vi "WT210 IEC 2015 Setup.vi"(0 "VISA Input":refnum<visa-resource-name>, 5 "V Range (6: 600V)":u16(ring)=4 items=["Auto", "15V", "30V", "60V", "150V", "300V", "600V"], 7 "A Range (12: 20A)":u16(ring)=10 items=["Auto", "5mA", "10mA", "20mA", "50mA", "100mA", "200mA", "0.5A", "1A", "2A", "5A", "10A", "20A", "50mV", "100mV", "200mV", "2.5V", "5V", "10V"], 11 "error in (no error)":errorcluster) -> (2 "VTHD":sgl format="%.3g", 4 "VISA Output":refnum<visa-resource-name>, 6 "Header File":string[][](array[string]), 15 "error out":errorcluster)   [LabVIEW 2016]
uses:
  <vilib>/Utility/error.llb/whitespace.ctl
  Yokogawa WT200 Series.lvlib
panel:
  in  "Tab Control":enum32{"Main", "Debug"}(tab)
  out "Sample Rate (1: 0.25s)":u16(ring)=1 items=["0.1s", "0.25s", "0.5s", "1s", "2s", "5s"]
  out "Sample Rate":string
  out "V Range":string
  out "A Range":string
  out "Instrument ID":string
  out "Date & Time":string
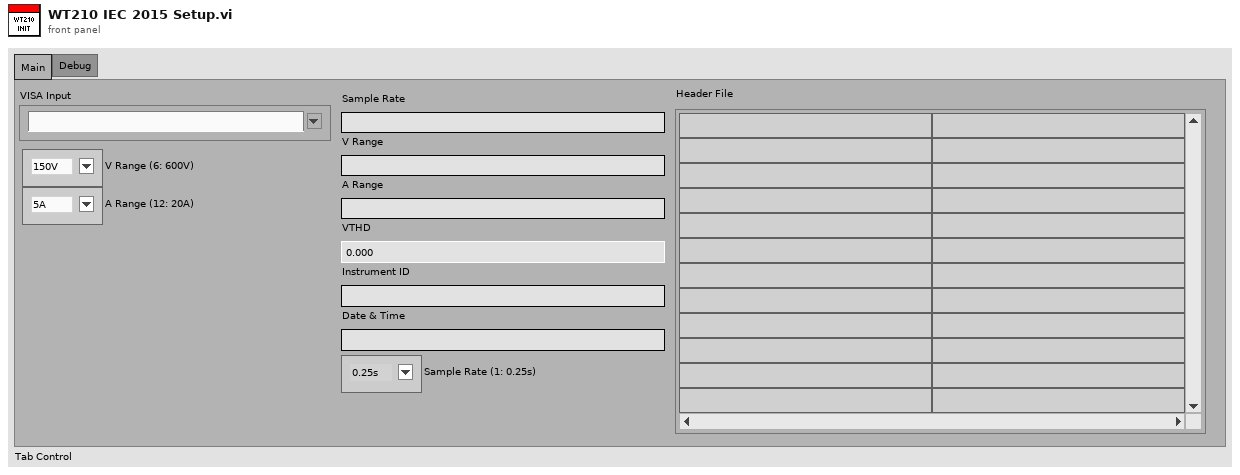
[diagram p1: front panel]
types:
  T1 = typedef "whitespace.ctl" = u16
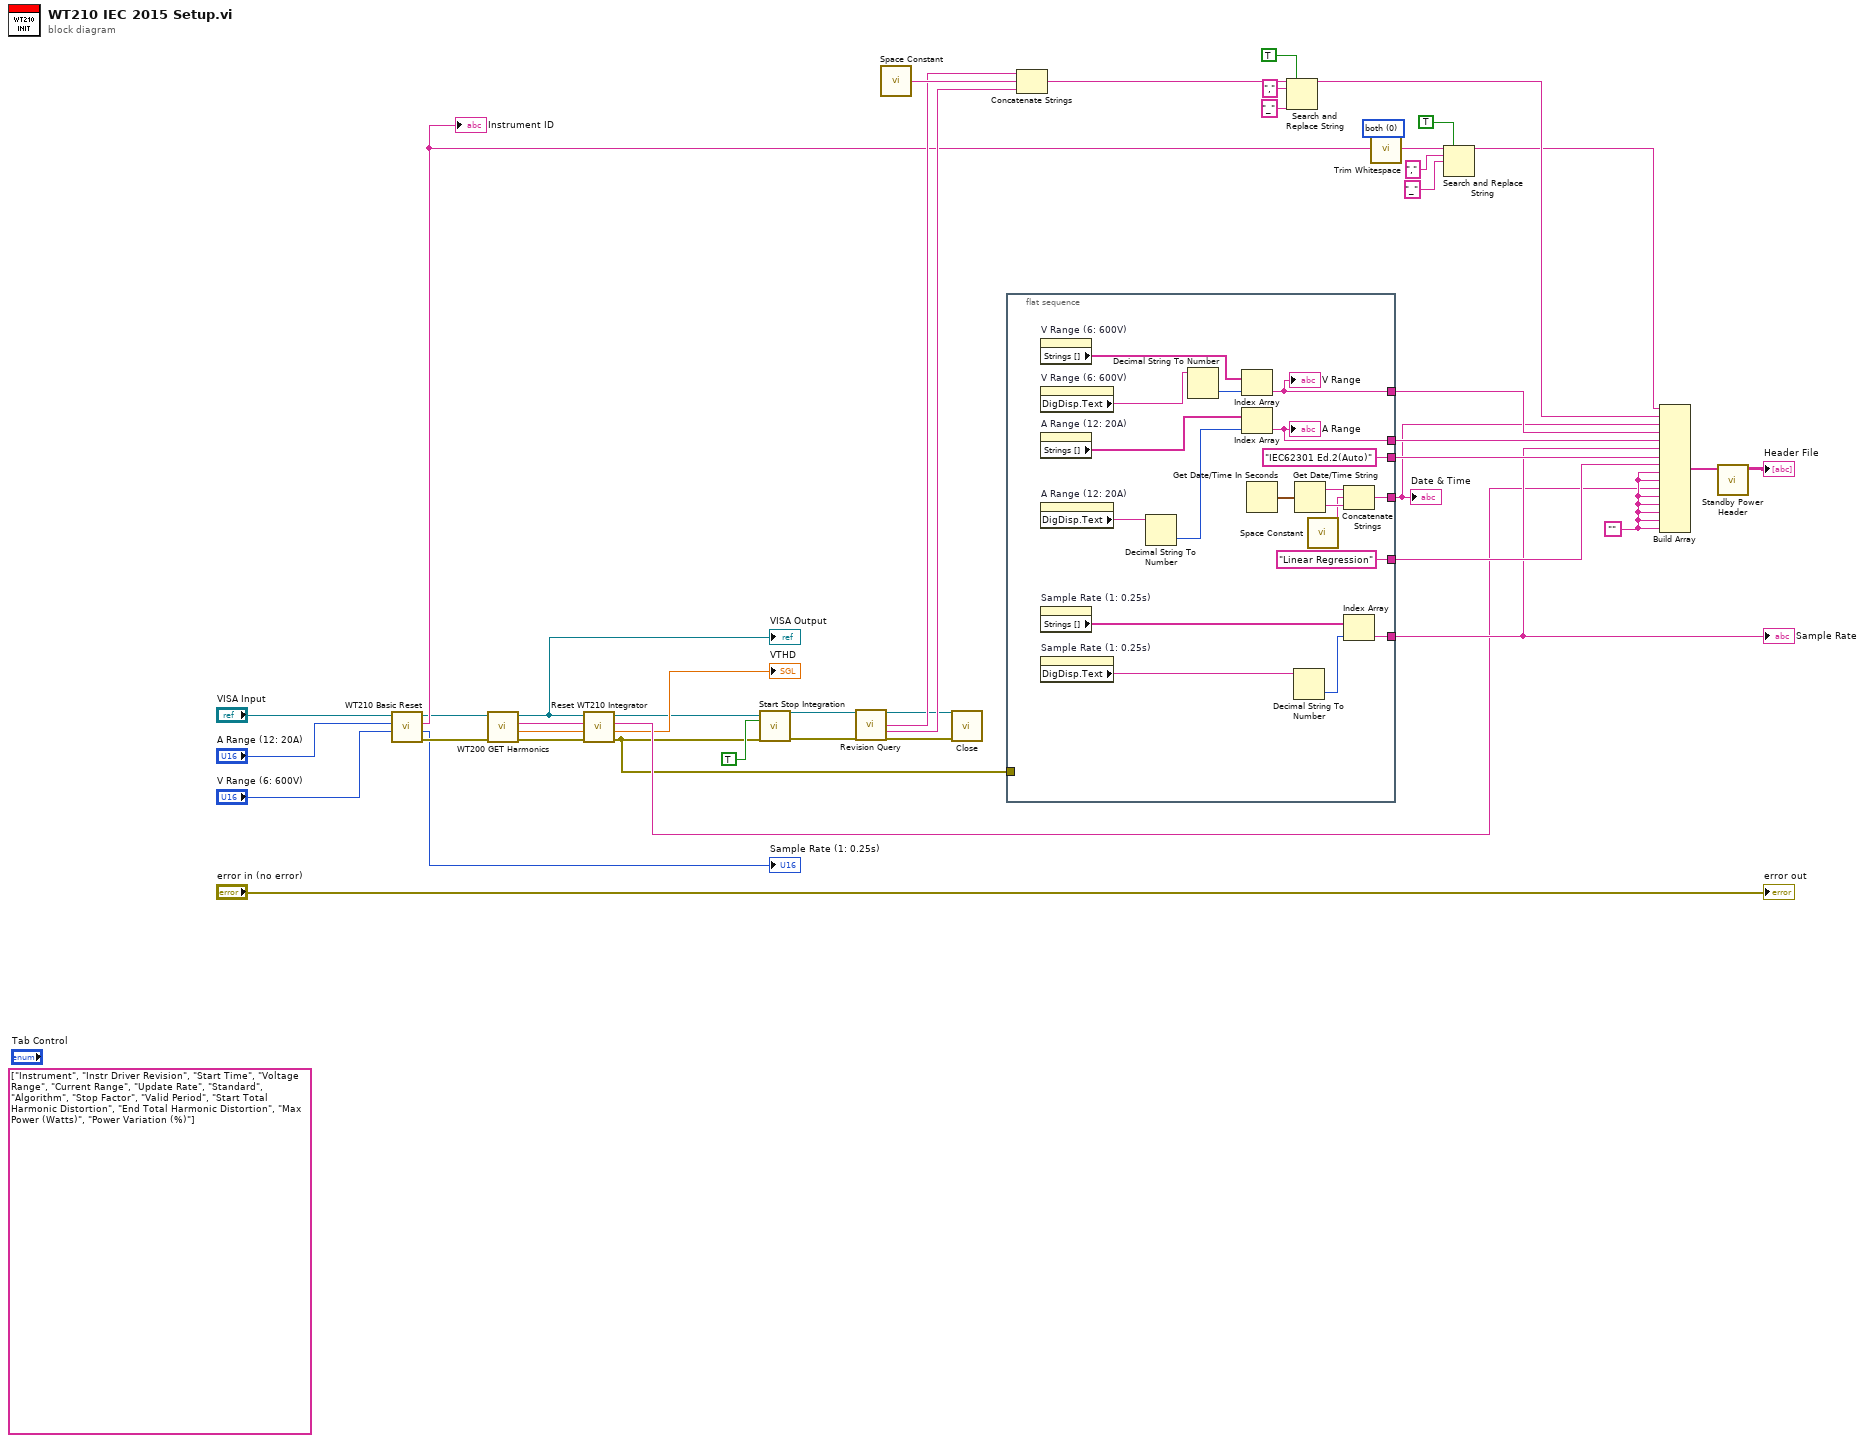
[diagram p0: block diagram]
diagram:
  w28 = T1 0 items=["both", "start of string", "end of string"] ("location (both)")
  w34 = ""
  (unwired) string[] ["Instrument", "Instr Driver Revision", "Start Time", "Voltage Range", "Current Range", "Update Rate", "Standard", "Algorithm", "Stop Factor", "Valid Period", "Start Total Harmonic Distortion", "End Total Harmonic Distortion", "Max Power (Watts)", "Power Variation (%)"]
  n1 = call "WT210 Basic Reset.vi"("V Range (6: 600V)"="V Range (6: 600V)", "A Range (12: 20A)"="A Range (12: 20A)", "VISA Refnum in"="VISA Input") -> ("error out"=w26:errorcluster, "Sample Rate (1: 0.25s)"=→"Sample Rate (1: 0.25s)":u16, "Instrument ID"=w29:string, "VISA Refnum out"=w27:refnum<visa-resource-name>)  [unwired: 5 in]
  "Instrument ID" <- w29
  n2 = call "WT200 GET Harmonics.vi"("error in (no error)"=w26, "VISA Refnum in"=w27) -> ("error out"=w10:errorcluster, "VTHD"=→"VTHD":dbl, "Final Harmonic Content U1"=w25:string, "VISA Refnum out"=w8:refnum<visa-resource-name>)  [unwired: 6 in]
  "VISA Output" <- w8
  n3 = call "Reset WT210 Integrator.vi"("error in (no error)"=w10, "VISA resource name"=w8) -> ("error out"=w9:errorcluster, "VISA resource name out"=w7:refnum<visa-resource-name>)  [unwired: 8 in]
  n4 = call "Start Stop Integration.vi"("VISA resource name"=w7, "Start/Stop (F: Stop)"=TRUE, "error in (no error)"=w9) -> ("VISA resource name out"=w5:refnum<visa-resource-name>, "error out"=w6:errorcluster)  [unwired: 11 in]
  n5 = call "Revision Query.vi"("VISA resource name"=w5, "error in (no error)"=w6) -> ("VISA resource name out"=w4:refnum<visa-resource-name>, "Instr Driver Revision"=w36:string, "Instr Firmware Revision"=w35:string, "error out"=w3:errorcluster)  [unwired: 10 in]
  n6 = call <vilib>:"Space Constant.vi"() -> ("String"=w37:string)
  n7 = call "Close.vi"("VISA resource name"=w4, "error in (no error)"=w3) -> ()  [unwired: 13 in, 1 out]
  n8 = flat-sequence {
    tunnel: [w55] -> w42
    tunnel: [w54] -> w41
    tunnel: ["IEC62301 Ed.2(Auto)" ("element")] -> w40
    tunnel: ["Linear Regression" ("element")] -> w39
    tunnel: w9 -> [_]
    tunnel: [w47] -> w33
    tunnel: [w43] -> w32
    frame #0 {
      n9 = property on="V Range (6: 600V)" class="Ring (strict)"() -> ("Strings []"=w59:string[])  [unwired: 2 in, 2 out]
      n10 = property on="V Range (6: 600V)" class="Ring (strict)"() -> ("DigDisp.Text"=w61:string)  [unwired: 2 in, 2 out]
      n11 = property on="A Range (12: 20A)" class="Ring (strict)"() -> ("Strings []"=w56:string[])  [unwired: 2 in, 2 out]
      n12 = property on="A Range (12: 20A)" class="Ring (strict)"() -> ("DigDisp.Text"=w58:string)  [unwired: 2 in, 2 out]
      n13 = property on="Sample Rate (1: 0.25s)" class="Ring (strict)"() -> ("Strings []"=w45:string[])  [unwired: 2 in, 2 out]
      n14 = property on="Sample Rate (1: 0.25s)" class="Ring (strict)"() -> ("DigDisp.Text"=w44:string)  [unwired: 2 in, 2 out]
      n15 = Decimal String To Number(string=w58) -> (number=w57:i32)  [unwired: 2 in, 1 out]
      n16 = Decimal String To Number(string=w61) -> (number=w60:i32)  [unwired: 2 in, 1 out]
      n17 = Index Array(array=w59, index=w60) -> (element=w55:string)
      "V Range" <- w55
      n18 = Index Array(array=w56, index=w57) -> (element=w54:string)
      "A Range" <- w54
      n19 = Get Date/Time In Seconds() -> (seconds since 1Jan1904=w48:timestamp)
      n20 = Decimal String To Number(string=w44) -> (number=w46:i32)  [unwired: 2 in, 1 out]
      n21 = Get Date/Time String(seconds (now)=w48) -> (date string=w50:string, time string=w51:string)  [unwired: 2 in]
      n22 = call <vilib>:"Space Constant.vi"() -> ("String"=w49:string)
      n23 = Concatenate Strings(w50, w49, w51) -> (w47:string)
      n24 = Index Array(array=w45, index=w46) -> (element=w43:string)
    }
  }
  n25 = Concatenate Strings(w36, w37, w35) -> (w18:string)
  n26 = Search and Replace String(replace all?=TRUE ("replace all? (F)"), input string=w18, search string=",", replace string="_" ("replace string (\"\")")) -> (result string=w17:string)  [unwired: 4 in, 3 out]
  n27 = call <vilib>:"Trim Whitespace.vi"("string"=w29, "location (both)"=w28) -> ("trimmed string"=w13:string)
  n28 = Search and Replace String(replace all?=TRUE ("replace all? (F)"), input string=w13, search string=",", replace string="_" ("replace string (\"\")")) -> (result string=w12:string)  [unwired: 4 in, 3 out]
  n29 = Build Array(w12, w17, w33, w42, w41, w32, w40, w39, w34, w34, w25, w34, w34, w34, w34, w34) -> (w23:string[])
  n30 = call "Standby Power Header.vi"("Array"=w23) -> ("Header File"=→"Header File":string[][])  [unwired: 9 in, 1 out]
  "error out" <- "error in (no error)"
  "Sample Rate" <- w32
  "Date & Time" <- w33
